vi "begin && file_int.vi"() -> ()   [LabVIEW 2012, in "LightPipes.lvlib"]
uses:
  LightPipes.lvlib
panel:
  in  "Initial Beam":path=path "C:/Users/Green Beret/Documents/Visual Studio 2012/Projects/LightPipes/LightPipes/lp12src/LabView/images/original/source.pgm"
  in  "Final Beam":path=path "C:/Users/Green Beret/Documents/Visual Studio 2012/Projects/LightPipes/LightPipes/lp12src/LabView/images/original/target_intensity.gpl"
  in  "c2":i16(ring) items=["subst", "mult"]
  in  "c1":i16(ring) items=["int", "pha"]
  out "field out":T1={"n_grid"=256, "@dummy control@"=0, "@dummy control@"=0, "@dummy control@"=0, "@dummy control@"=0, "size"=0.01, "lambda"=1e-06, "int1"=0, "int2"=0, "int3"=0, "@dummy control@"=0, "@dummy control@"=0, "@dummy control@"=0, "@dummy control@"=0, "double1"=0.0, "double2"=0.0, "double3"=0.0, "real"=300089408, "imaginary"=314572864}
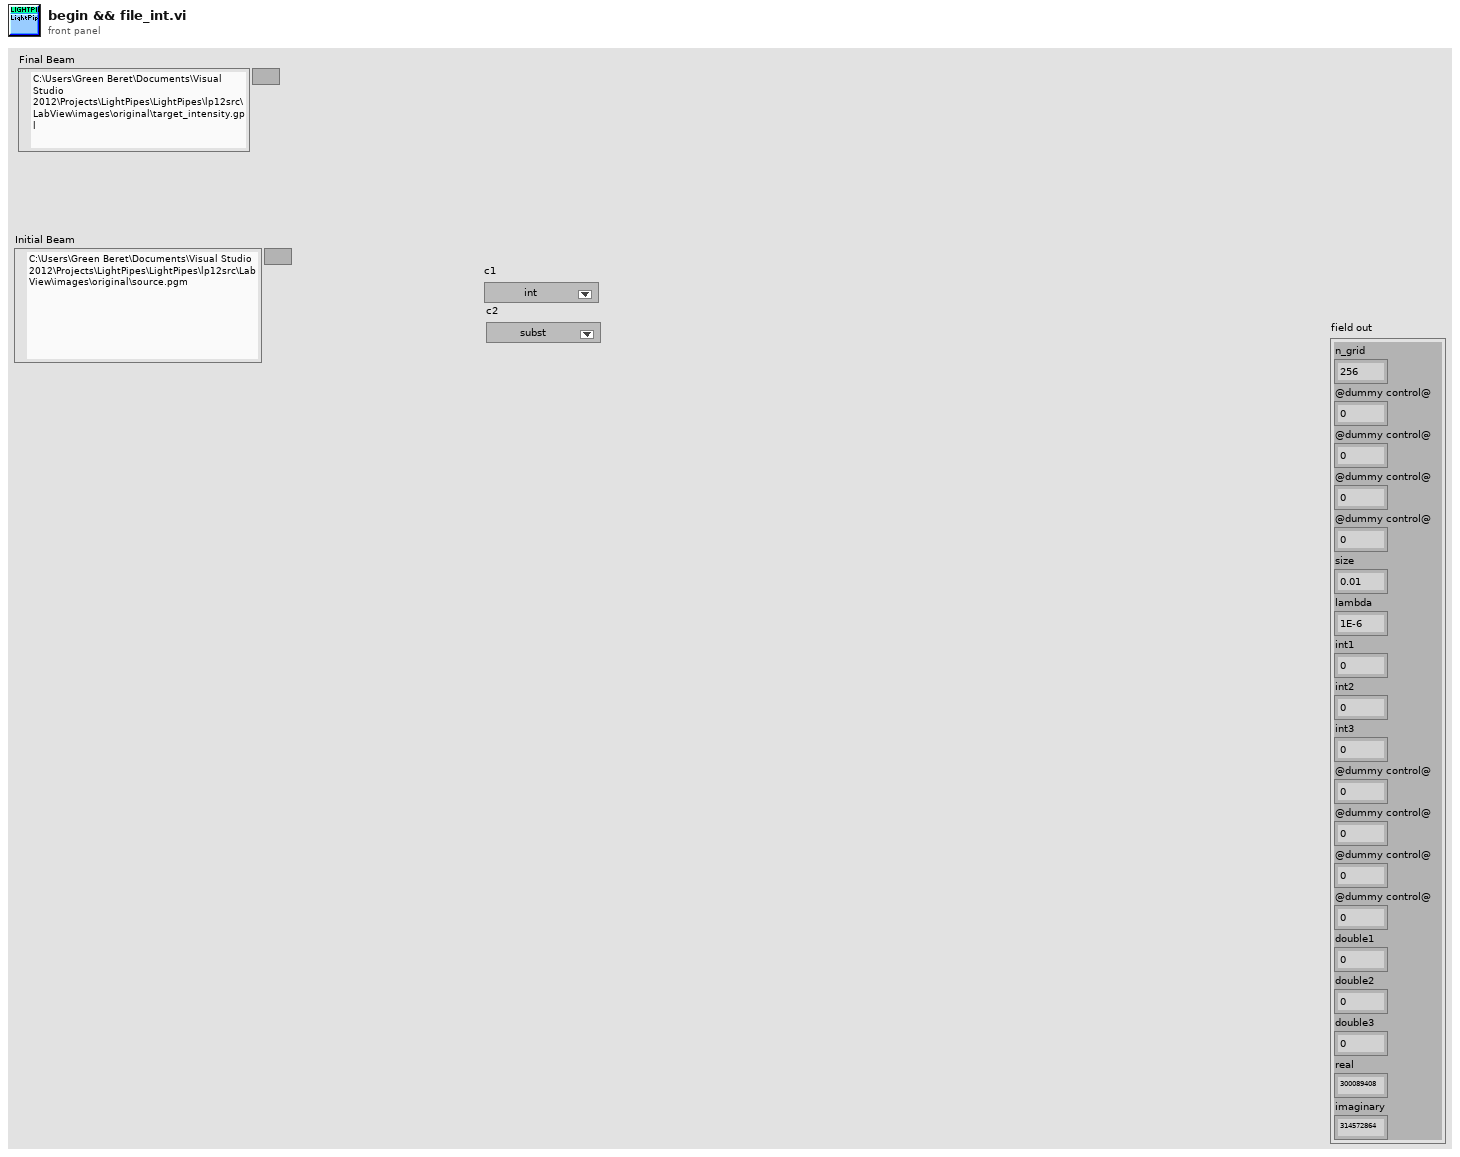
[diagram p1: front panel]
types:
  T1 = cluster{"n_grid":i32, "@dummy control@":i8, "@dummy control@":i8, "@dummy control@":i8, "@dummy control@":i8, "size":dbl, "lambda":dbl, "int1":i32, "int2":i32, "int3":i32, "@dummy control@":i8, "@dummy control@":i8, "@dummy control@":i8, "@dummy control@":i8, "double1":dbl, "double2":dbl, "double3":dbl, "real":u32, "imaginary":u32}
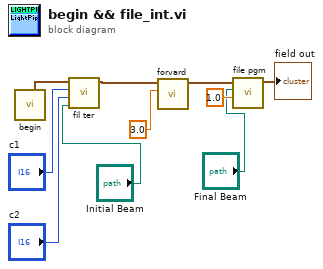
[diagram p0: block diagram]
diagram:
  n1 = call "begin.vi"() -> ("field out"=w7:T1)  [unwired: 11 in]
  n2 = call "fil ter.vi"("Path"="Initial Beam", "multiplication/ substitution"="c2", "intensity / phase"="c1", "field"=w7) -> ("field out"=w4:T1)  [unwired: 6 in, 1 out]
  n3 = call "forvard.vi"("distance"=3.0, "field"=w4) -> ("field out"=w9:T1)  [unwired: 9 in]
  n4 = call "file pgm.vi"("gamma"=1.0, "Path"="Final Beam", "field"=w9) -> ("field out"=→"field out":T1)  [unwired: 7 in, 1 out]
